vi "全局变量.vi"() -> ()   [LabVIEW 2017]
panel:
  out "启用问号":bool
  out "雷数":i32
  in  "难度":enum16{"初级", "中级", "高级"}(ring)
  out "列数":i32
  out "行数":i32
  out "面板边界":cluster{"左":i32, "上":i32, "右":i32, "下":i32}
  out "错误音乐":path
  out "跟随音乐":path
  out "胜利音乐":path
  out "失败音乐":path
  out "扩展音乐":path
  out "循环计时":bool
  out "地雷":i16[][](array[numeric])
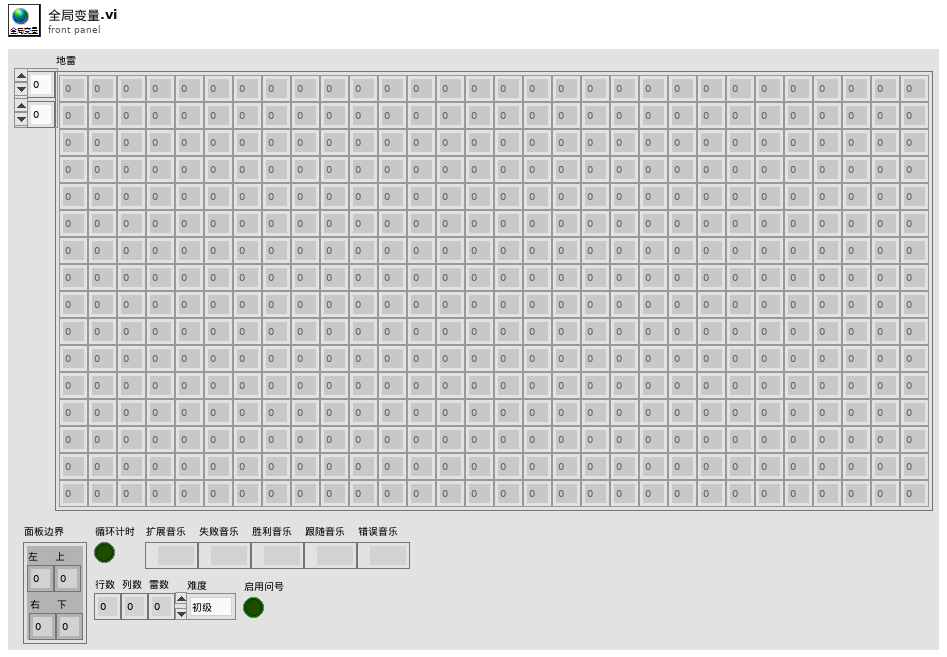
[diagram p1: front panel]
diagram:
